vi "Data File Processing UI.vi"() -> ()   [LabVIEW 2011]
doc: "This example shows how to create a built-in user interface (UI) in the Microphone Array Startup (MAS). You can create such a UI basing on the template named ma_analysis template.vi. Refer to <B>Example 3: Create a Simple UI</B> part in the Software Description of MAS for more information."
uses:
  sub VIs/Data File Processing UI_ChannelSet.ctl
  sub VIs/Data File Processing UI Message Type Define.ctl
  sub VIs/Data File Processing UI_GlobalData.ctl
panel:
  out "Exit":bool
  in  "Return":bool
  in  "Save Project":bool
  in  "Open Project":bool
  out "Graph":dbl[][](graph)
  in  "SelectAll":bool
  in  "ChSetArray":T1[](array[typedef])
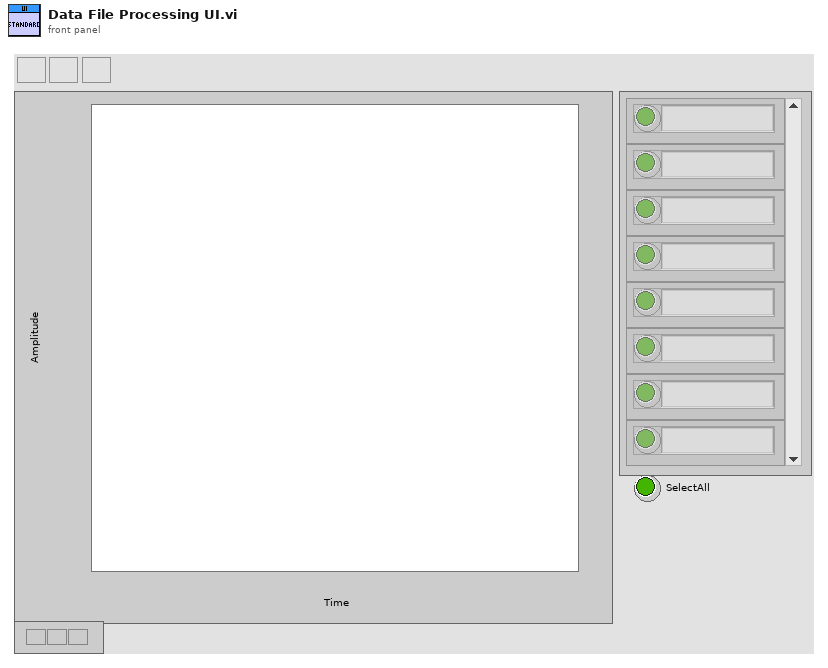
[diagram p1: front panel]
types:
  T1 = typedef "Data File Processing UI_ChannelSet.ctl" = cluster{"Select":bool, "Channel":string}
  T2 = typedef "Data File Processing UI_GlobalData.ctl" = cluster{"error":errorcluster, "CurrentFilePath":path, "File Start Time":dbl, "File End Time":dbl}
  T3 = typedef "Data File Processing UI Message Type Define.ctl" = enum32{"Initialize", "SleepThread", "ErrorHandler", "NoEvent", "PreExit", "Exit", "----Action----", "OpenFile", "SaveFile", "RedrawGraph", "SelectChannel"}
  T4 = typedef "Data File Processing UI Message Define.ctl" = cluster{"data":variant, "type":T3}
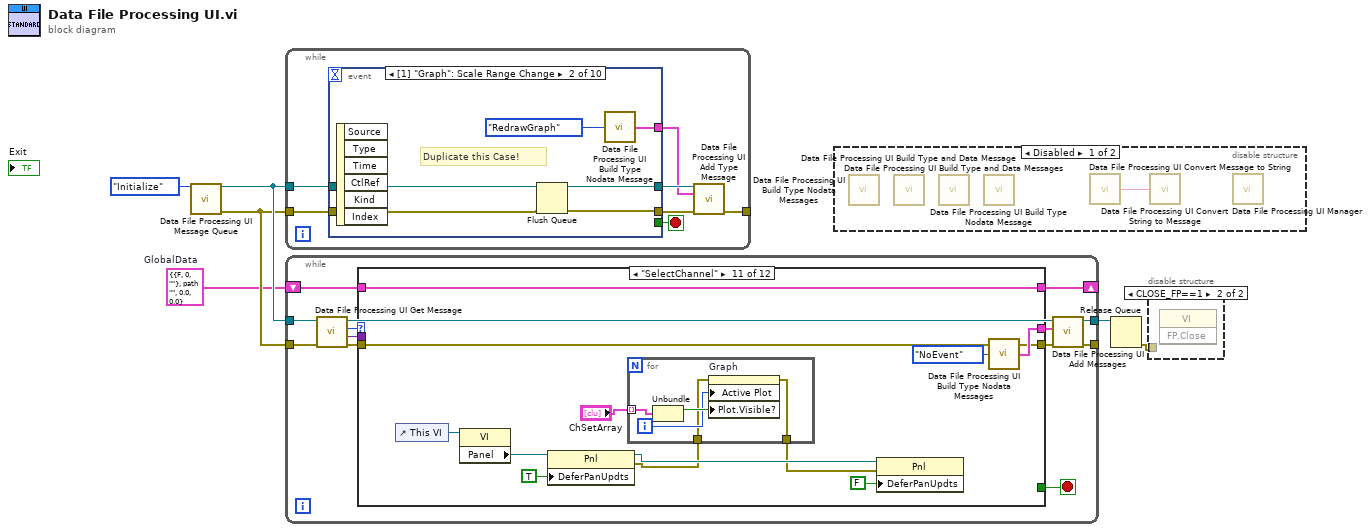
[diagram p0: block diagram]
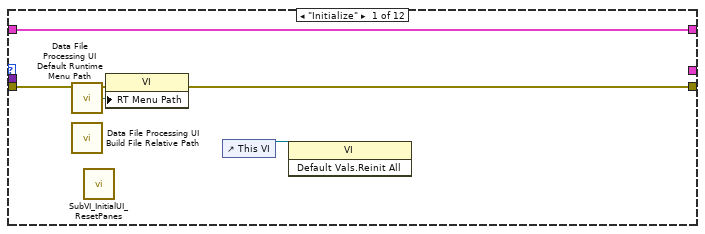
[diagram p4: hidden frame]
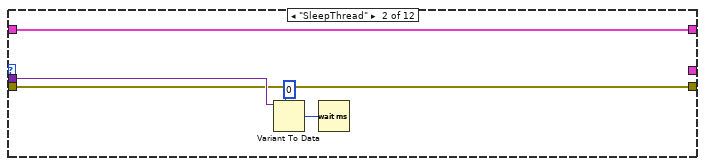
[diagram p5: hidden frame]
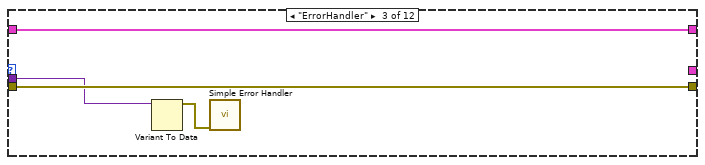
[diagram p6: hidden frame]
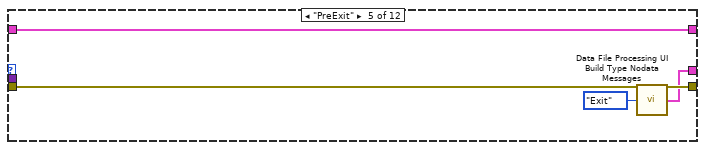
[diagram p8: hidden frame]
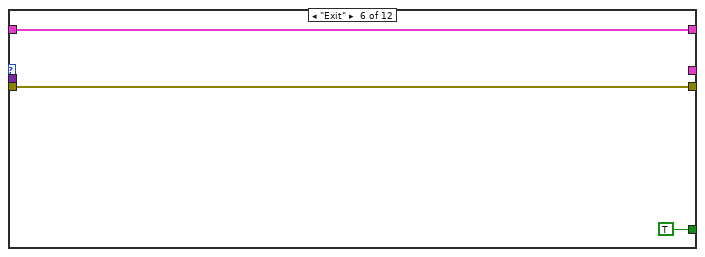
[diagram p9: hidden frame]
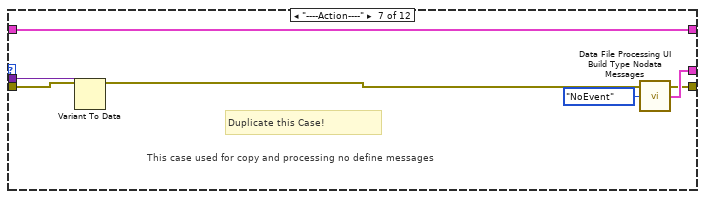
[diagram p10: hidden frame]
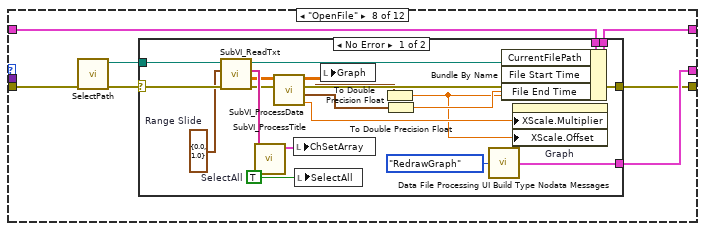
[diagram p11: hidden frame]
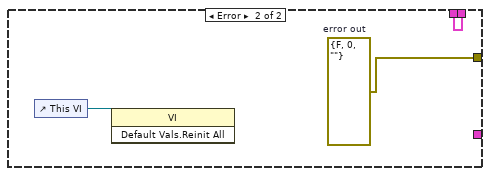
[diagram p12: hidden frame]
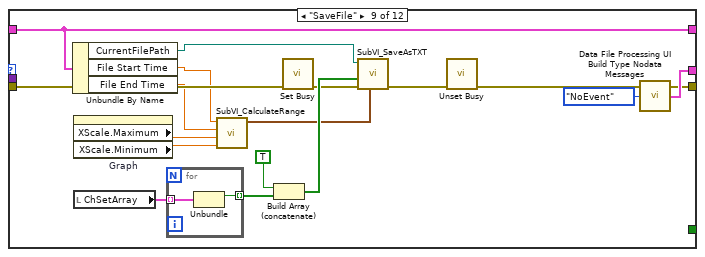
[diagram p13: hidden frame]
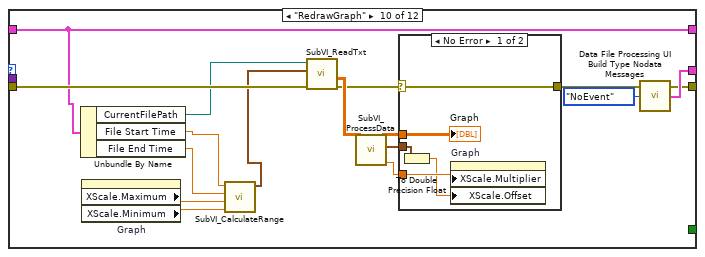
[diagram p14: hidden frame]
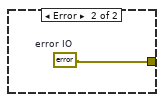
[diagram p15: hidden frame]
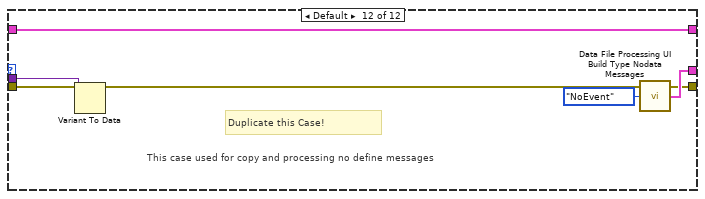
[diagram p16: hidden frame]
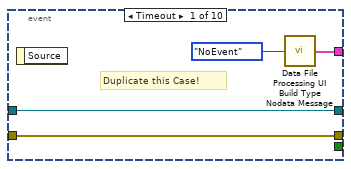
[diagram p17: hidden frame]
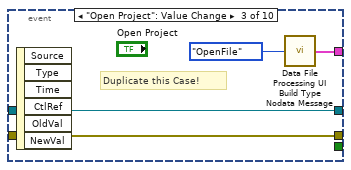
[diagram p18: hidden frame]
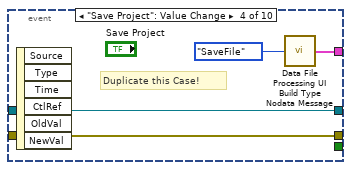
[diagram p19: hidden frame]
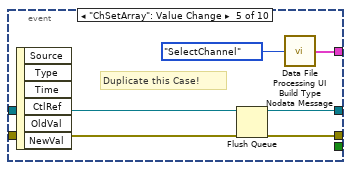
[diagram p20: hidden frame]
diagram:
  w1 = T2 {"error"={"status"=FALSE, "code"=0, "source"=""}, "CurrentFilePath"=path "", "File Start Time"=0.0, "File End Time"=0.0}  # GlobalData
  n1 = call "Data File Processing UI Message Queue.vi"("msg type"=Data_File_Processing_UI_Message_Type_Define."Initialize") -> ("queue out"=w5:refnum<queue>, "error out"=w4:errorcluster)  [unwired: 13 in]
  n2 = while {
    tunnel: w5 -> [w13]
    tunnel: w4 -> [w12]
    tunnel: [w8] -> _
    stop <- w11 stop-if-true
    n3 = event shown="[1] \"Graph\": Scale Range Change" {
      selector: _ -> [_ _ _ _ _ _ _ _ _ _]
      dyn-events: _ -> [_ _ _ _ _ _ _ _ _ _]
      timeout: _ -> [_ _ _ _ _ _ _ _ _ _]
      tunnel: w13 -> [w17 w23 w27 w31 w36 w44 w51 w54 w67 w75]
      tunnel: [w17 w20 w27 w31 w32 w40 w51 w54 w67 w75] -> w10
      tunnel: w12 -> [w16 w19 w26 w30 w35 w43 w50 w57 w66 w74]
      tunnel: [w16 w18 w26 w30 w35 w43 w50 w57 w66 w74] -> w9
      tunnel: [_ _ _ _ _ _ _ w53 TRUE TRUE] -> w11
      tunnel: [w14 w21 w24 w28 w33 w41 w48 w52 w65 w72] -> w7
      event Timeout {
        # "Duplicate this Case!"
        n4 = event-data() -> ()  [unwired: 2 out]
        n5 = call "Data File Processing UI Build Type Nodata Message.vi"("type"=Data_File_Processing_UI_Message_Type_Define."NoEvent" ("Msg")) -> ("msg out"=w14:T4)  [unwired: 14 out]
      }
      event "Graph": Scale Range Change {
        # "Duplicate this Case!"
        n6 = event-data() -> ()  [unwired: 7 out]
        n7 = Flush Queue(queue=w23, error in (no error)=w19) -> (queue out=w20:refnum<queue>, error out=w18:errorcluster)  [unwired: 1 out]
        n8 = call "Data File Processing UI Build Type Nodata Message.vi"("type"=Data_File_Processing_UI_Message_Type_Define."RedrawGraph" ("Msg")) -> ("msg out"=w21:T4)  [unwired: 14 out]
      }
      event "Open Project": Value Change {
        # "Duplicate this Case!"
        n9 = event-data() -> ()  [unwired: 7 out]
        n10 = call "Data File Processing UI Build Type Nodata Message.vi"("type"=Data_File_Processing_UI_Message_Type_Define."OpenFile" ("Msg")) -> ("msg out"=w24:T4)  [unwired: 14 out]
      }
      event "Save Project": Value Change {
        # "Duplicate this Case!"
        n11 = event-data() -> ()  [unwired: 7 out]
        n12 = call "Data File Processing UI Build Type Nodata Message.vi"("type"=Data_File_Processing_UI_Message_Type_Define."SaveFile" ("Msg")) -> ("msg out"=w28:T4)  [unwired: 14 out]
      }
      event "ChSetArray": Value Change {
        # "Duplicate this Case!"
        n13 = event-data() -> ()  [unwired: 7 out]
        n14 = Flush Queue(queue=w36) -> (queue out=w32:refnum<queue>)  [unwired: 1 in, 2 out]
        n15 = call "Data File Processing UI Build Type Nodata Message.vi"("type"=Data_File_Processing_UI_Message_Type_Define."SelectChannel" ("Msg")) -> ("msg out"=w33:T4)  [unwired: 14 out]
      }
      event "SelectAll": Value Change {
        n16 = event-data() -> ()  [unwired: 7 out]
        n17 = local read "ChSetArray"() -> (w37:T1[])
        n18 = for {
          tunnel: w37 -> [w47] mode=indexing
          tunnel: [w46] -> w38 mode=indexing
          tunnel: "SelectAll" -> [w45]
          n19 = Bundle By Name(cluster=w47, "Select"=w45) -> (w46:T1)
        }
        n20 = Flush Queue(queue=w44) -> (queue out=w40:refnum<queue>)  [unwired: 1 in, 2 out]
        n21 = local write "ChSetArray"(w38) -> ()
        n22 = call "Data File Processing UI Build Type Nodata Message.vi"("type"=Data_File_Processing_UI_Message_Type_Define."SelectChannel" ("Msg")) -> ("msg out"=w41:T4)  [unwired: 14 out]
      }
      event Panel Resize {
        n23 = event-data() -> ()  [unwired: 8 out]
        n24 = call "Data File Processing UI Build Type Nodata Message.vi"("type"=Data_File_Processing_UI_Message_Type_Define."NoEvent" ("Msg")) -> ("msg out"=w48:T4)  [unwired: 14 out]
      }
      event Menu Selection (User) {
        n25 = event-data() -> ("ItemTag"=w56:string, "ItemPath"=w55:string)  [unwired: 1 out]
        n26 = case shown="\"EXIT\"" w56 {
          tunnel: w55 -> [_ _]
          tunnel: [_ TRUE] -> w53
          tunnel: [w59 w61] -> w52
          frame Default {
            # "Duplicate this Case!"
            n27 = call "Data File Processing UI Build Type Nodata Message.vi"("type"=Data_File_Processing_UI_Message_Type_Define."NoEvent" ("Msg")) -> ("msg out"=w59:T4)  [unwired: 14 out]
          }
          frame "EXIT" {
            n28 = call "Data File Processing UI Build Type Nodata Message.vi"("type"=Data_File_Processing_UI_Message_Type_Define."PreExit" ("Msg")) -> ("msg out"=w61:T4)  [unwired: 14 out]
          }
        }
      }
      event Panel Close? {
        n29 = event-data() -> ()  [unwired: 2 out]
        n30 = event-data("Discard?"=TRUE) -> ()  [unwired: 1 in, 1 out]
        n31 = call "Data File Processing UI Build Type Nodata Message.vi"("type"=Data_File_Processing_UI_Message_Type_Define."PreExit" ("Msg")) -> ("msg out"=w65:T4)  [unwired: 14 out]
      }
      event "Return": Value Change {
        n32 = event-data() -> ()  [unwired: 7 out]
        n33 = Not(x="Return") -> (.not. x?=w69:bool)
        n34 = property on="Return" class="Bool (strict)"("Value"=w69) -> ()  [unwired: 2 in, 2 out]
        n35 = call "Data File Processing UI Build Type Nodata Message.vi"("type"=Data_File_Processing_UI_Message_Type_Define."PreExit" ("Msg")) -> ("msg out"=w72:T4)  [unwired: 14 out]
      }
    }
    n36 = call "Data File Processing UI Add Type Message.vi"("queue in"=w10, "Msg"=w7, "error in"=w9) -> ("error out"=w8:errorcluster)  [unwired: 12 out]
  }
  n37 = while {
    shift-right: [w86] -> _
    shift-left: w1 -> [w87]
    tunnel: w5 -> [w81]
    tunnel: [w76] -> w6
    tunnel: w4 -> [w82]
    tunnel: [w80] -> _
    stop <- w88 stop-if-true
    n38 = call "Data File Processing UI Get Message.vi"("error in"=w82, "msg queue in"=w81) -> ("error out"=w85:errorcluster, "data"=w84:variant, "msg"=w83:T3, "msg queue out"=w78:refnum<queue>)  [unwired: 6 out]
    n39 = case shown="\"SelectChannel\"" w83 {
      tunnel: [_ _ _ _ _ TRUE _ _ _ _ _ _] -> w88
      tunnel: [w90 w97 w102 w104 w108 w110 w112 w119 w153 w172 w195 w204] -> w79
      tunnel: w85 -> [w91 w97 w102 w104 w108 w110 w112 w118 w156 w179 w195 w204]
      tunnel: w87 -> [w93 w96 w101 w103 w107 w109 w113 w122 w147 w167 w196 w205]
      tunnel: [w93 w96 w101 w103 w107 w109 w113 w120 w147 w167 w196 w205] -> w86
      tunnel: [_ _ _ _ w106 _ w115 w123 w162 w180 w198 w207] -> w77
      tunnel: w84 -> [_ w98 w99 _ _ _ w116 _ _ _ _ w208]
      frame "Initialize" {
        n40 = call "Data File Processing UI Default Runtime Menu Path.vi"() -> ("runtime menu path"=w92:path)  [unwired: 15 in]
        n41 = call "Data File Processing UI Build File Relative Path.vi"() -> ()  [unwired: 15 in, 1 out]
        n42 = call "SubVI_InitialUI_ResetPanes.vi"() -> ()  [unwired: 12 in]
        n43 = property class="VI"(error in=w91, "RT Menu Path"=w92) -> (error out=w90:errorcluster)  [unwired: 1 in, 1 out]
        n44 = control-ref of="This VI"() -> (w89:refnum<vi>)
        n45 = invoke class="VI" method="Default Vals.Reinit All"(reference=w89) -> ()  [unwired: 2 in, 3 out]
      }
      frame "SleepThread" {
        n46 = Variant To Data(type=u32 0 ("milliseconds to wait"), Variant=w98) -> (data=w94:u32)  [unwired: 1 in, 1 out]
        n47 = Wait (ms)(milliseconds to wait=w94) -> ()  [unwired: 1 out]
      }
      frame "ErrorHandler" {
        n48 = Variant To Data(Variant=w99) -> (data=w100:errorcluster)  [unwired: 2 in, 1 out]
        n49 = call <vilib>:"Simple Error Handler.vi"("error in (no error)"=w100) -> ()  [unwired: 1 in, 8 out]
      }
      frame "NoEvent" {
      }
      frame "PreExit" {
        n50 = call "Data File Processing UI Build Type Nodata Messages.vi"("type"=Data_File_Processing_UI_Message_Type_Define."Exit") -> ("msg out"=w106:T4[])  [unwired: 14 out]
      }
      frame "Exit" {
      }
      frame "----Action----" {
        # "Duplicate this Case!"
        # "This case used for copy and processing no define messages"
        n51 = Variant To Data(type=w112, Variant=w116) -> ()  [unwired: 1 in, 2 out]
        n52 = call "Data File Processing UI Build Type Nodata Messages.vi"("type"=Data_File_Processing_UI_Message_Type_Define."NoEvent") -> ("msg out"=w115:T4[])  [unwired: 14 in]
      }
      frame "OpenFile" {
        n53 = call "SelectPath.vi"("error in (no error)"=w118) -> ("error out"=w117:errorcluster, "selected path"=w121:path)  [unwired: 9 in]
        n54 = case shown="No Error" w117 {
          selector: w117 -> [w132 _]
          tunnel: [w142 _] -> w123
          tunnel: w122 -> [w140 w145]
          tunnel: w121 -> [w139 _]
          tunnel: [w138 w145] -> w120
          tunnel: [w134 w144] -> w119
          frame No Error {
            w133 = TRUE  # SelectAll
            w131 = cluster{dbl, dbl} {0.0, 1.0}  # Range Slide
            n55 = call "SubVI_ReadTxt.vi"("error in"=w132, "Range Slide"=w131, "file path (use dialog)"=w139) -> ("error out"=w134:errorcluster, "Data Array"=w127:dbl[][], "Title"=w136:string[], "path"=w137:path)  [unwired: 5 in]
            n56 = call "SubVI_ProcessTitle.vi"("Title"=w136) -> ("Array"=w135:T1[])  [unwired: 10 in]
            n57 = call "SubVI_ProcessData.vi"("Data Array"=w127) -> ("dt"=w125:dbl, "end time stamp"=w129:timestamp, "start time stamp"=w130:timestamp, "Data Array out"=w126:dbl[][])  [unwired: 7 in]
            n58 = local write "ChSetArray"(w135) -> ()
            n59 = local write "SelectAll"(w133) -> ()
            n60 = local write "Graph"(w126) -> ()
            n61 = To Double Precision Float(number=w130) -> (double precision float=w124:dbl)
            n62 = To Double Precision Float(number=w129) -> (double precision float=w128:dbl)
            n63 = call "Data File Processing UI Build Type Nodata Messages.vi"("type"=Data_File_Processing_UI_Message_Type_Define."RedrawGraph") -> ("msg out"=w142:T4[])  [unwired: 14 in]
            n64 = Bundle By Name(cluster=w140, "CurrentFilePath"=w137, "File Start Time"=w124, "File End Time"=w128) -> (w138:T2)
            n65 = property on="Graph" class="WFGraph (strict)"("XScale.Multiplier"=w125, "XScale.Offset"=w124) -> ()  [unwired: 2 in, 2 out]
          }
          frame Error {
            w144 = errorcluster {"status"=FALSE, "code"=0, "source"=""}  # error out
            n66 = control-ref of="This VI"() -> (w143:refnum<vi>)
            n67 = invoke class="VI" method="Default Vals.Reinit All"(reference=w143) -> ()  [unwired: 2 in, 3 out]
          }
        }
      }
      frame "SaveFile" {
        n68 = Unbundle By Name(w147) -> ("CurrentFilePath"=w148:path, "File Start Time"=w149:dbl, "File End Time"=w151:dbl)
        n69 = property on="Graph" class="WFGraph (strict)"() -> ("XScale.Maximum"=w152:dbl, "XScale.Minimum"=w150:dbl)  [unwired: 2 in, 2 out]
        n70 = local read "ChSetArray"() -> (w160:T1[])
        n71 = for {
          tunnel: w160 -> [w164] mode=indexing
          tunnel: [w163] -> w158 mode=indexing
          n72 = Unbundle(w164) -> ("Select"=w163:bool)  [unwired: 1 out]
        }
        n73 = call "SubVI_CalculateRange.vi"("XScale.Minimum"=w150, "XScale.Maximum"=w152, "File End Time"=w151, "File Start Time"=w149) -> ("Range"=w146:cluster{dbl, dbl})  [unwired: 7 in]
        n74 = Build Array (concatenate)(TRUE, w158) -> (w157:bool[])
        n75 = call <vilib>:"Set Busy.vi"("error in (no error)"=w156) -> ("error out"=w155:errorcluster)  [unwired: 9 in, 1 out]
        n76 = call "SubVI_SaveAsTXT.vi"("Range Slide"=w146, "error in"=w155, "Channel Selection"=w157, "source file path"=w148) -> ("error out"=w154:errorcluster)  [unwired: 7 in]
        n77 = call <vilib>:"Unset Busy.vi"("error in (no error)"=w154) -> ("error out"=w153:errorcluster)  [unwired: 10 in]
        n78 = call "Data File Processing UI Build Type Nodata Messages.vi"("type"=Data_File_Processing_UI_Message_Type_Define."NoEvent") -> ("msg out"=w162:T4[])  [unwired: 14 in]
      }
      frame "RedrawGraph" {
        n79 = Unbundle By Name(w167) -> ("CurrentFilePath"=w166:path, "File Start Time"=w168:dbl, "File End Time"=w170:dbl)
        n80 = property on="Graph" class="WFGraph (strict)"() -> ("XScale.Maximum"=w171:dbl, "XScale.Minimum"=w169:dbl)  [unwired: 2 in, 2 out]
        n81 = call "SubVI_CalculateRange.vi"("XScale.Minimum"=w169, "XScale.Maximum"=w171, "File End Time"=w170, "File Start Time"=w168) -> ("Range"=w165:cluster{dbl, dbl})  [unwired: 7 in]
        n82 = call "SubVI_ReadTxt.vi"("error in"=w179, "Range Slide"=w165, "file path (use dialog)"=w166) -> ("error out"=w176:errorcluster, "Data Array"=w178:dbl[][])  [unwired: 5 in, 2 out]
        n83 = call "SubVI_ProcessData.vi"("Data Array"=w178) -> ("dt"=w175:dbl, "start time stamp"=w174:timestamp, "Data Array out"=w177:dbl[][])  [unwired: 7 in, 1 out]
        n84 = case shown="No Error" w176 {
          selector: w176 -> [w184 _]
          tunnel: w177 -> [w185 _]
          tunnel: [w184 w186] -> w172
          tunnel: w175 -> [w183 _]
          tunnel: w174 -> [w182 _]
          frame No Error {
            n85 = To Double Precision Float(number=w182) -> (double precision float=w181:dbl)
            n86 = property on="Graph" class="WFGraph (strict)"("XScale.Multiplier"=w183, "XScale.Offset"=w181) -> ()  [unwired: 2 in, 2 out]
            "Graph" <- w185
          }
          frame Error {
            w186 = errorcluster {"status"=FALSE, "code"=0, "source"=""}  # error IO
          }
        }
        n87 = call "Data File Processing UI Build Type Nodata Messages.vi"("type"=Data_File_Processing_UI_Message_Type_Define."NoEvent") -> ("msg out"=w180:T4[])  [unwired: 14 in]
      }
      frame "SelectChannel" {
        n88 = control-ref of="This VI"() -> (w191:refnum<vi>)
        n89 = property class="VI"(reference=w191) -> ("Panel"=w192:refnum<vi>)  [unwired: 1 in, 2 out]
        n90 = property class="Pnl"(reference=w192, "DeferPanUpdts"=TRUE ("Defer Panel Updates")) -> (reference out=w189:refnum<vi>, error out=w188:errorcluster)  [unwired: 1 in]
        n91 = for {
          tunnel: "ChSetArray" -> [w203] mode=indexing
          tunnel: w188 -> [w200]
          tunnel: [w199] -> w187
          i -> [w201]
          n92 = Unbundle(w203) -> ("Select"=w202:bool)  [unwired: 1 out]
          n93 = property on="Graph" class="WFGraph (strict)"(error in=w200, "Active Plot"=w201, "Plot.Visible?"=w202) -> (error out=w199:errorcluster)  [unwired: 1 in, 1 out]
        }
        n94 = property class="Pnl"(reference=w189, error in=w187, "DeferPanUpdts"=FALSE ("Defer Panel Updates")) -> ()  [unwired: 2 out]
        n95 = call "Data File Processing UI Build Type Nodata Messages.vi"("type"=Data_File_Processing_UI_Message_Type_Define."NoEvent") -> ("msg out"=w198:T4[])  [unwired: 14 in]
      }
      frame Default {
        # "Duplicate this Case!"
        # "This case used for copy and processing no define messages"
        n96 = Variant To Data(type=w204, Variant=w208) -> ()  [unwired: 1 in, 2 out]
        n97 = call "Data File Processing UI Build Type Nodata Messages.vi"("type"=Data_File_Processing_UI_Message_Type_Define."NoEvent") -> ("msg out"=w207:T4[])  [unwired: 14 in]
      }
    }
    n98 = call "Data File Processing UI Add Messages.vi"("error in"=w79, "messages"=w77, "msg queue in"=w78) -> ("error out"=w80:errorcluster, "msg queue out"=w76:refnum<queue>)  [unwired: 7 out]
  }
  n99 = disable-structure shown="Disabled" {
    frame Disabled {
      n100 = call "Data File Processing UI Build Type Nodata Messages.vi"() -> ()  [unwired: 15 in, 1 out]
      n101 = call "Data File Processing UI Build Type and Data Message.vi"() -> ()  [unwired: 15 in, 1 out]
      n102 = call "Data File Processing UI Build Type and Data Messages.vi"() -> ()  [unwired: 15 in, 1 out]
      n103 = call "Data File Processing UI Build Type Nodata Message.vi"() -> ()  [unwired: 15 in, 1 out]
      n104 = call "Data File Processing UI Convert Message to String.vi"() -> ("msg"=w209:string)  [unwired: 15 in]
      n105 = call "Data File Processing UI Convert String to Message.vi"("msg in"=w209) -> ()  [unwired: 14 in, 1 out]
      n106 = call "Data File Processing UI Manager.vi"() -> ()  [unwired: 12 in]
    }
    frame Enabled {
    }
  }
  n107 = Release Queue(queue=w6) -> (error out=w2:errorcluster)  [unwired: 1 in, 3 out]
  n108 = disable-structure shown="CLOSE_FP==1" {
    disable-tunnel: w2 -> [_ _]
    frame condition #0 (active) {
    }
    frame condition #1 {
      n109 = invoke class="VI" method="FP.Close"() -> ()  [unwired: 3 in, 3 out]
    }
  }
